vi "Example XYGraph Peaks&Valleys.vi"() -> ()   [LabVIEW 2020]
uses:
  controls/PeaksValleyOptions.ctl
  Graph Extensions.lvlib
panel:
  in  "Peaks and Valleys":T1={"Peaks"={"#"=3, "size"=8, "WidthThreshold"=3, "AmplitudeThreshold"=0.0, "Fill"=TRUE, "PlotIndexes (All)"=[]}, "Valleys"={"#"=3, "size"=7, "WidthThreshold"=3, "AmplitudeThreshold"=0.0, "Fill"=TRUE, "PlotIndexes (All)"=[]}} {"Valleys"."AmplitudeThreshold" min=0.0 format="%.3f"; "Valleys"."WidthThreshold" min=3; "Valleys"."size" min=1 max=50; "Peaks"."AmplitudeThreshold" min=0.0 format="%.3f"; "Peaks"."WidthThreshold" min=3; "Peaks"."size" min=1 max=50}
  out "XY Graph":cluster{dbl[], dbl[]}[](graph)
  # "Instructions: Adjust any of the options at the right. to see the effect."
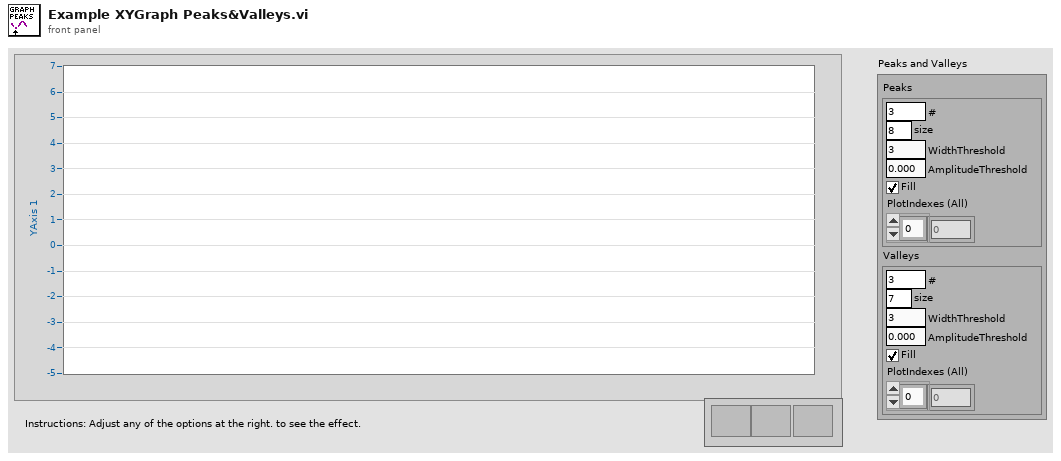
[diagram p1: front panel]
types:
  T1 = typedef "Graph Extensions.lvlib/PeaksValleyOptions.ctl" = cluster{"Peaks":cluster{"#":i32, "size":i16, "WidthThreshold":i32, "AmplitudeThreshold":dbl, "Fill":bool, "PlotIndexes (All)":u16[]}, "Valleys":cluster{"#":i32, "size":i16, "WidthThreshold":i32, "AmplitudeThreshold":dbl, "Fill":bool, "PlotIndexes (All)":u16[]}}
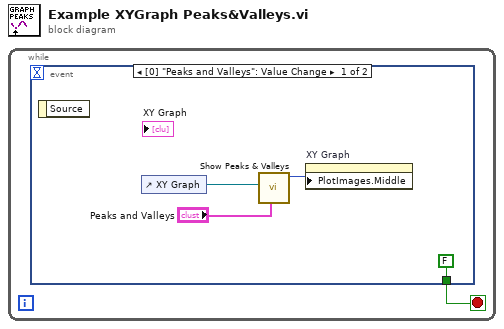
[diagram p0: block diagram]
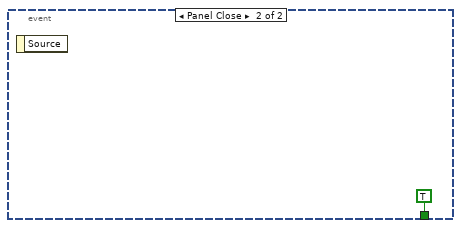
[diagram p2: hidden frame]
diagram:
  n1 = while {
    stop <- w1 stop-if-true
    n2 = event shown="[0] \"Peaks and Valleys\": Value Change" {
      selector: _ -> [_ _]
      dyn-events: _ -> [_ _]
      timeout: _ -> [_ _]
      tunnel: [FALSE TRUE] -> w1
      event Value Change {
        n3 = event-data() -> ()  [unwired: 1 in, 1 out]
        n4 = control-ref of="XY Graph"() -> (w2:refnum<vi>)
        n5 = call "Show Peaks & Valleys.vi"("peaksValleysOptions"="Peaks and Valleys", "XY Graph"=w2) -> ("output picture"=w3:picture)  [unwired: 8 in, 1 out]
        n6 = property on="XY Graph" class="XYGraph (strict)"("PlotImages.Middle"=w3) -> ()  [unwired: 2 in, 2 out]
      }
      event Panel Close {
        n7 = event-data() -> ()  [unwired: 1 in, 1 out]
      }
    }
  }
